vi "LabOneHandIn.vi"() -> ()   [LabVIEW 2024]
panel:
  in  "stop":bool
  out "Volume Indicator":dbl format="%_4f"
  out "Height Indicator":dbl(slide) scale=0.0..10.0
  in  "Height Control":dbl(slide) scale=0.0..10.0
  out "Indicator 2":dbl(slide) scale=0.0..100.0
  in  "Control 2":dbl(knob) scale=0.0..10.0
  out "Status":bool
  in  "Switch 2":bool
  in  "Switch 1":bool
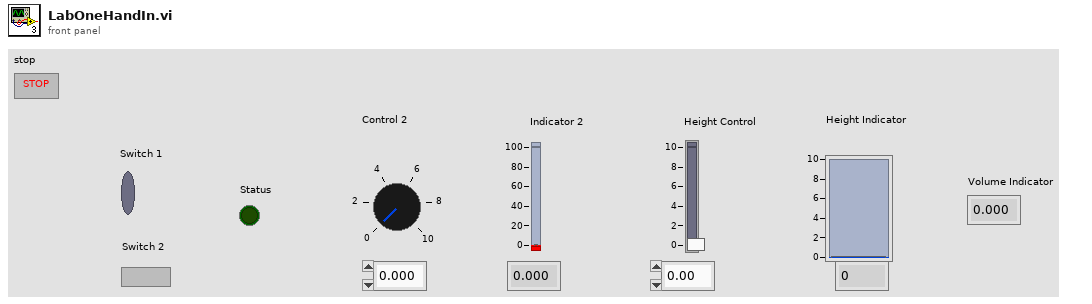
[diagram p1: front panel]
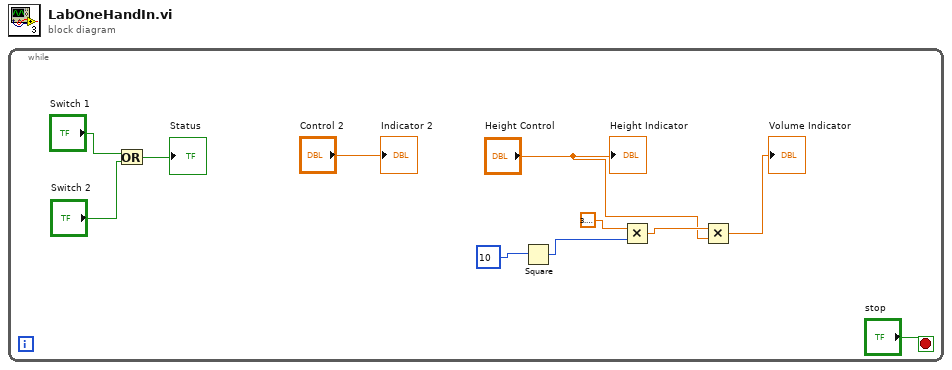
[diagram p0: block diagram]
diagram:
  n1 = while {
    stop <- "stop" stop-if-true
    n2 = Or(x="Switch 1", y="Switch 2") -> (x .or. y?=→"Status":bool)
    n3 = Square(x=10) -> (x^2=w3:i32)
    n4 = Multiply(x=3.141592653589793, y=w3) -> (x*y=w7:dbl)
    n5 = Multiply(x=w7, y="Height Control") -> (x*y=→"Volume Indicator":dbl)
    "Indicator 2" <- "Control 2"
    "Height Indicator" <- "Height Control"
  }
